vi "ToTable.vi"(8 "error in (no error)":errorcluster, 9 "Table Index":i32, 10 "variant":variant, 11 "node in":refnum<class "control module editor.lvclass">) -> (0 "error out":errorcluster, 1 "row header":string[](array[string]), 2 "table":string[][](array[string]), 3 "node in out":refnum<class "control module editor.lvclass">)   [LabVIEW 2013, in "control module editor.lvclass"]
doc: "Copyright 2015 National Instruments Corporation\n\nLicensed under the Apache License, Version 2.0 (the \"License\"); you may not use this file except in compliance with the License. You may obtain a copy of the License at http://www.apache.org/licenses/LICENSE-2.0\nUnless required by applicable law or agreed to in writing, software distributed under the License is distributed on an \"AS IS\" BASIS, WITHOUT WARRANTIES OR CONDITIONS OF ANY KIND, either express or implied. See the License for the specific language governing permissions and limitations under the License."
uses:
  control module editor.lvclass
  configuration/control module configuration.lvclass
  <vilib>/NI/Module Execution Interface/Engine Configuration/engine configuration.lvclass
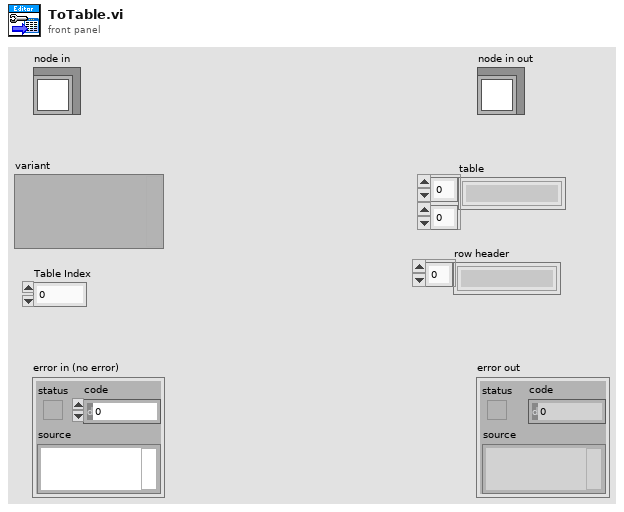
[diagram p1: front panel]
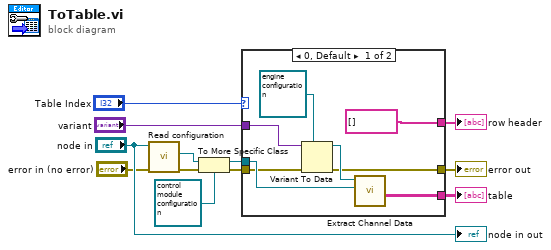
[diagram p0: block diagram]
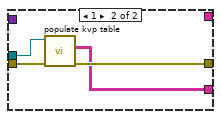
[diagram p2: hidden frame]
diagram:
  n1 = call-dynamic "Read configuration.vi"("error in"="error in (no error)", "NISE_CEF_serializable node in"="node in") -> ("error out"=w4:errorcluster, "configuration"=w11:refnum<class "NISE_CEF_serializable configuration.lvclass">)  [unwired: 7 in, 1 out]
  n2 = To More Specific Class(target class=refnum<class "control module configuration.lvclass"> refnum ("fixed channel configuration"), reference=w11, error in=w4) -> (specific class reference=w9:refnum<class "control module configuration.lvclass">, error out=w3:errorcluster)
  n3 = case shown="0, Default" "Table Index" {
    tunnel: w9 -> [w16 w24]
    tunnel: [w15 w21] -> w8
    tunnel: [string[] [] ("row header") _] -> w6
    tunnel: w3 -> [w14 w23]
    tunnel: [w13 w22] -> w2
    tunnel: "variant" -> [w18 _]
    frame 0, Default {
      n4 = Variant To Data(error in=w14, type=refnum<class "engine configuration.lvclass"> refnum ("Engine Configuration"), Variant=w18) -> (data=w17:refnum<class "engine configuration.lvclass">, error out=w13:errorcluster)
      n5 = call "Extract Channel Data.vi"("module configuration in"=w16, "Engine Configuration"=w17) -> ("Channel Data"=w15:string[][])  [unwired: 9 in]
    }
    frame 1 {
      n6 = call "populate kvp table.vi"("error in"=w23, "fixed channel configuration in"=w24) -> ("error out"=w22:errorcluster, "kvp's"=w21:string[][])  [unwired: 7 in, 1 out]
    }
  }
  "error out" <- w2
  "table" <- w8
  "row header" <- w6
  "node in out" <- "node in"
